vi "285A_RelMove.vi"(7 "VISA资源名称":refnum<visa-resource-name>, 8 "error in (no error)":errorcluster caption="错误输入（无错误）", 9 "Z 2":dbl, 10 "Y 2":dbl, 11 "X 2":dbl) -> (0 "error out":errorcluster caption="错误输出", 1 "read buffer 2":string, 2 "read buffer":string, 3 "VISA resource name out 2":refnum<visa-resource-name>, 4 "read buffer 4":string, 6 "Serial Settings:Number of Bytes at Serial Port 2":u32)   [LabVIEW 2016]
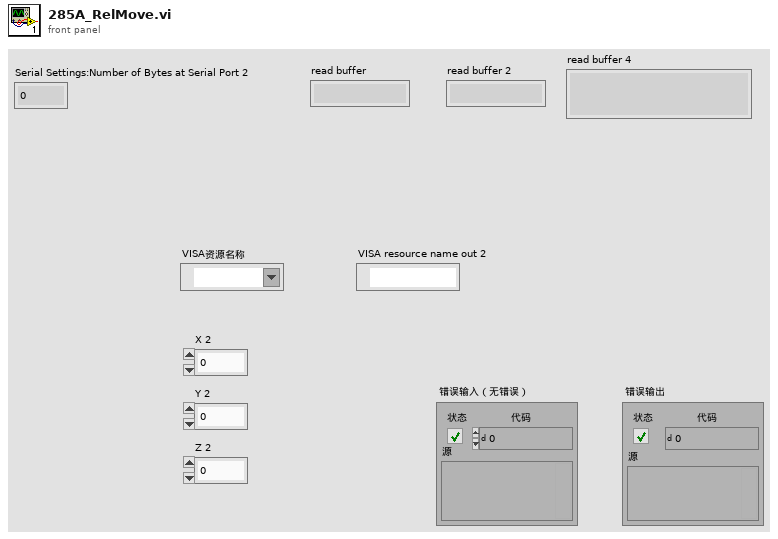
[diagram p1: front panel]
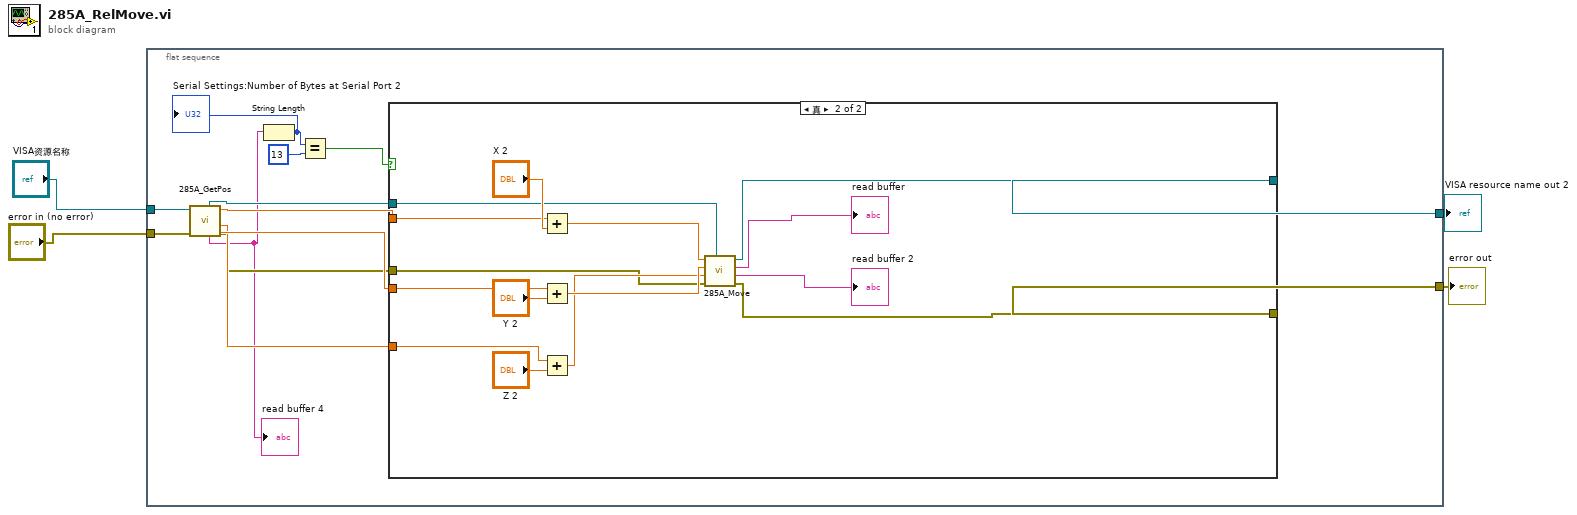
[diagram p0: block diagram]
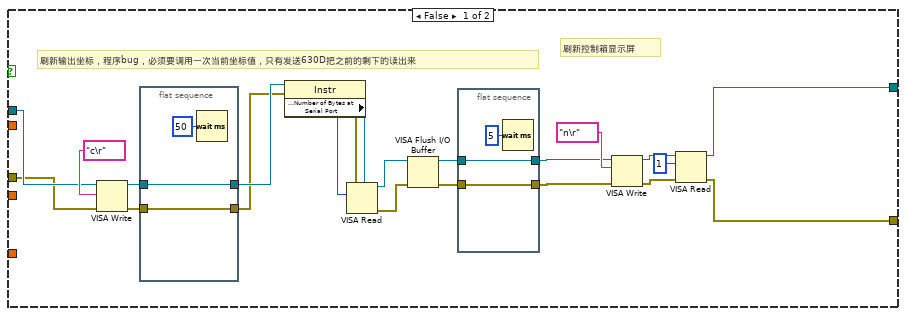
[diagram p2: hidden frame]
diagram:
  n1 = flat-sequence {
    tunnel: "VISA资源名称" -> [w16]
    tunnel: "error in (no error)" -> [w15]
    tunnel: [w8] -> w2
    tunnel: [w7] -> w1
    frame #0 {
      n2 = call "285A_GetPos.vi"("error in (no error)"=w15, "VISA资源名称"=w16) -> ("error out"=w9:errorcluster, "Z"=w11:dbl, "Y"=w12:dbl, "X"=w13:dbl, "read buffer"=w6:string, "VISA资源名称输出"=w10:refnum<visa-resource-name>)  [unwired: 4 in]
      "read buffer 4" <- w6
      n3 = String Length(string=w6) -> (length=w5:i32)
      "Serial Settings:Number of Bytes at Serial Port 2" <- w5
      n4 = Equal?(x=w5, y=13) -> (x = y?=w14:bool)
      n5 = case shown="真" w14 {
        tunnel: [w19 w50] -> w8
        tunnel: [w18 w49] -> w7
        tunnel: w13 -> [_ w57]
        tunnel: w12 -> [_ w56]
        tunnel: w11 -> [_ w55]
        tunnel: w10 -> [w23 w51]
        tunnel: w9 -> [w22 w48]
        frame False {
          # "刷新输出坐标，程序bug，必须要调用一次当前坐标值，只有发送630D把之前的剩下的读出来"
          # "刷新控制箱显示屏"
          n6 = VISA Write ("VISA写入")(VISA resource name=w23, write buffer="c\r" ("写入缓冲区"), error in (no error)=w22) -> (VISA resource name out=w27:refnum<visa-resource-name>, error out=w26:errorcluster)  [unwired: 1 out]
          n7 = flat-sequence {
            tunnel: w27 -> [w41]
            tunnel: w26 -> [w40]
            tunnel: [w41] -> w25
            tunnel: [w40] -> w24
            frame #0 {
              n8 = Wait (ms)(milliseconds to wait=u32 50 ("等待时间（毫秒）")) -> ()  [unwired: 1 out]
            }
          }
          n9 = property class="Instr"(reference=w25, error in=w24) -> (reference out=w30:refnum<visa-resource-name>, error out=w31:errorcluster, "Serial Settings:Number of Bytes at Serial Port"=w29:u32)
          n10 = VISA Read(VISA resource name=w30, byte count=w29, error in (no error)=w31) -> (VISA resource name out=w21:refnum<visa-resource-name>, error out=w20:errorcluster)  [unwired: 2 out]
          n11 = VISA Flush I/O Buffer(VISA resource name=w21, error in (no error)=w20) -> (VISA resource name out=w38:refnum<visa-resource-name>, error out=w37:errorcluster)  [unwired: 1 in]
          n12 = flat-sequence {
            tunnel: w38 -> [w44]
            tunnel: w37 -> [w43]
            tunnel: [w44] -> w36
            tunnel: [w43] -> w35
            frame #0 {
              n13 = Wait (ms)(milliseconds to wait=u32 5 ("等待时间（毫秒）")) -> ()  [unwired: 1 out]
            }
          }
          n14 = VISA Write ("VISA写入")(VISA resource name=w36, write buffer="n\r" ("写入缓冲区"), error in (no error)=w35) -> (VISA resource name out=w34:refnum<visa-resource-name>, error out=w33:errorcluster)  [unwired: 1 out]
          n15 = VISA Read(VISA resource name=w34, byte count=u32 1 ("字节总数"), error in (no error)=w33) -> (VISA resource name out=w19:refnum<visa-resource-name>, error out=w18:errorcluster)  [unwired: 2 out]
        }
        frame True {
          n16 = Add(x=w57, y="X 2") -> (x+y=w54:dbl)
          n17 = Add(x=w56, y="Y 2") -> (x+y=w53:dbl)
          n18 = Add(x=w55, y="Z 2") -> (x+y=w52:dbl)
          n19 = call "285A_Move.vi"("VISA resource name out"=w51, "error in (no error)"=w48, "Abso_Z"=w52, "Abso_Y"=w53, "Abso_X"=w54) -> ("error out"=w49:errorcluster, "read buffer 2"=→"read buffer 2":string, "read buffer"=→"read buffer":string, "VISA resource name out 2"=w50:refnum<visa-resource-name>)  [unwired: 3 in]
        }
      }
    }
  }
  "error out" <- w1
  "VISA resource name out 2" <- w2
